vi "Resize Graph.vi"(11 "Intensity Graph Reference":refnum<vi>) -> ()   [LabVIEW 2015]
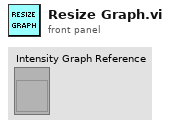
[diagram p1: front panel]
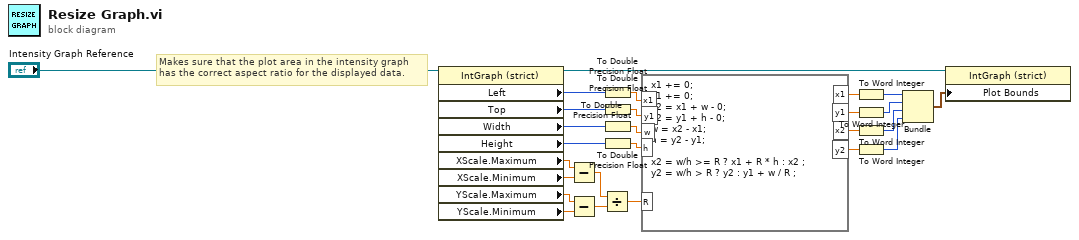
[diagram p0: block diagram]
diagram:
  # "Makes sure that the plot area in the intensity graph\nhas the correct aspect ratio for the displayed data."
  n1 = property class="IntGraph (strict)"(reference="Intensity Graph Reference") -> (reference out=w18:refnum<vi>, "Left"=w26:i32, "Top"=w25:i32, "Width"=w24:u32, "Height"=w23:u32, "XScale.Maximum"=w7:dbl, "XScale.Minimum"=w6:dbl, "YScale.Maximum"=w5:dbl, "YScale.Minimum"=w4:dbl)  [unwired: 1 in, 1 out]
  n2 = Subtract(x=w7, y=w6) -> (x-y=w3:dbl)
  n3 = Subtract(x=w5, y=w4) -> (x-y=w2:dbl)
  n4 = Divide(x=w3, y=w2) -> (x/y=w8:dbl)
  n5 = To Double Precision Float(number=w26) -> (double precision float=w16:dbl)
  n6 = To Double Precision Float(number=w25) -> (double precision float=w15:dbl)
  n7 = To Double Precision Float(number=w24) -> (double precision float=w14:dbl)
  n8 = To Double Precision Float(number=w23) -> (double precision float=w13:dbl)
  n9 = formula code="x1 += 0;\ny1 += 0;\nx2 = x1 + w - 0;\ny2 = y1 + h - 0;\nw = x2 - x1;\nh = y2 - y1;\n\nx2 = w/h >= R ? x1 + R * h : x2 ;\ny2 = w/h > R ? y2 : y1 + w / R ;"("x1"=w16, "y1"=w15, "w"=w14, "h"=w13, "R"=w8) -> ("x1"=w21:dbl, "y1"=w22:dbl, "x2"=w20:dbl, "y2"=w19:dbl)
  n10 = To Word Integer(number=w21) -> (16bit integer=w12:i16)
  n11 = To Word Integer(number=w22) -> (16bit integer=w11:i16)
  n12 = To Word Integer(number=w20) -> (16bit integer=w10:i16)
  n13 = To Word Integer(number=w19) -> (16bit integer=w9:i16)
  n14 = Bundle(w12, w11, w10, w9) -> (w17:cluster{i16, i16, i16, i16})  [unwired: 1 in]
  n15 = property class="IntGraph (strict)"(reference=w18, "Plot Bounds"=w17) -> ()  [unwired: 1 in, 2 out]
